vi "pf Get Camera Property Int.vi"(8 "error in (no error)":errorcluster, 10 "pProperty":string, 11 "iPort":i32) -> (0 "error out":errorcluster, 3 "function return":i32)   [LabVIEW 2025, in "Photonfocus_Toolkit.lvlib"]
doc: "PFCONFIG_API int pfGetCameraPropertyI(const char* pProperty);"
uses:
  Photonfocus_Toolkit.lvlib
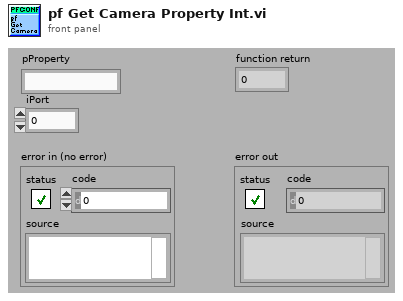
[diagram p1: front panel]
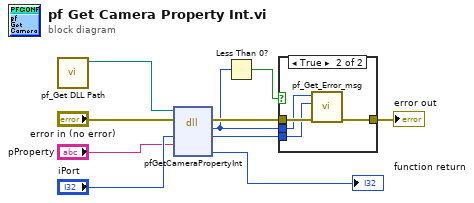
[diagram p0: block diagram]
diagram:
  n1 = call "pf_Get DLL Path.vi"() -> ("DLL path"=w9:path)  [unwired: 1 in, 10 out]
  n2 = dll-call lib="S:/Progetti/Photonfocus/Codice/DEV/PFConfig_lvlib/PFConfig.*" fn="pfGetCameraPropertyInt"(path in=w9, error in="error in (no error)", "iPort"="iPort", "pProperty"="pProperty") -> (error out=w8:errorcluster, "return type"=w2:i32, "iPort"=w1:i32, "value"=→"function return":i32)  [unwired: 2 in, 2 out]
  n3 = Less Than 0?(x=w2) -> (x < 0?=w3:bool)
  n4 = case shown="True" w3 {
    tunnel: w8 -> [w11 w15]
    tunnel: [w11 w14] -> w7
    tunnel: w2 -> [_ w13]
    tunnel: w1 -> [_ w12]
    frame False {
    }
    frame True {
      n5 = call "pf_Get_Error_msg.vi"("error in (no error)"=w15, "iPort"=w12, "error code"=w13) -> ("error out"=w14:errorcluster)  [unwired: 8 out]
    }
  }
  "error out" <- w7
